vi "fomula 노드로 C언어로 버블솔트 구현.vi"() -> ()   [LabVIEW 2025]
panel:
  out "output variable":dbl[](array[numeric])
  in  "input variable":dbl[](array[numeric])
  # "이건 열값이라 1차원 배열도 있어서 sizeOfDim(a, 0) 행열 이렇게 크기구는듯"
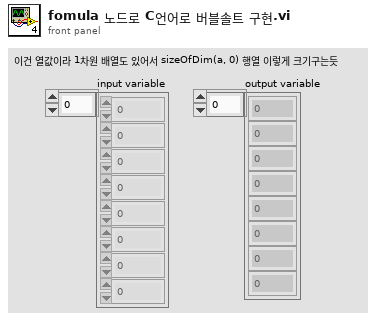
[diagram p1: front panel]
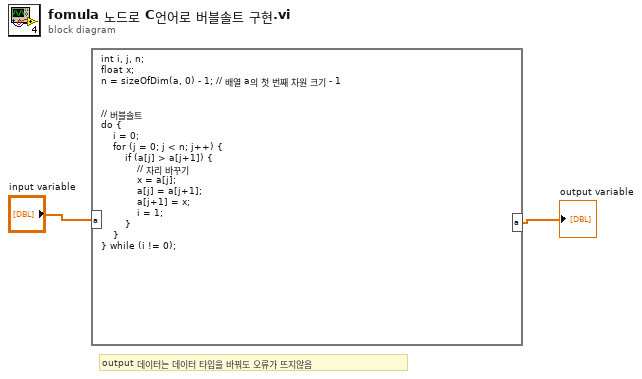
[diagram p0: block diagram]
diagram:
  # "output 데이터는 데이터 타입을 바꿔도 오류가 뜨지않음"
  n1 = formula code="int i, j, n;\nfloat x;\nn = sizeOfDim(a, 0) - 1; // 배열 a의 첫 번째 차원 크기 - 1\n\n\n// 버블솔트\ndo {\n    i = 0;  \n    for (j = 0; j < n; j++) {\n        if (a[j] > a[j+1]) {\n            // 자리 바꾸기\n            x = a[j];\n            a[j] = a[j+1];\n            a[j+1] = x;\n            i = 1;  \n        }\n    }\n} while (i != 0);"("a"="input variable") -> ("a"=→"output variable":dbl[])
